vi "GLdrv_FILE_DRIVE.vi"(0 "Connection ID":T1, 11 "error in (no error)":errorcluster) -> (4 "Connection ID Out":T1, 6 "Drive out":string[](array[string]), 15 "error out":errorcluster)   [LabVIEW 2017, in "GL860_Driver.lvlib"]
doc: "認識されているデバイスを表示します\nMEM=内蔵メモリ\nSD=SDカード\n例) :FILE:DRIVE “MEM:HDD SD:HDD”"
uses:
  GL860_Driver.lvlib
  ConnectionID.ctl
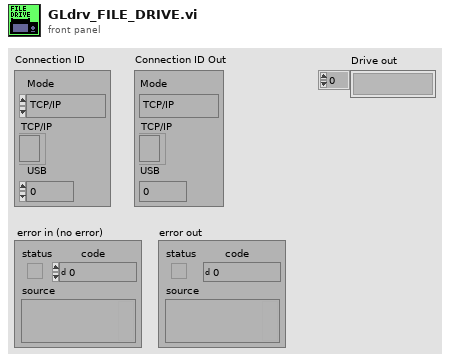
[diagram p1: front panel]
types:
  T1 = typedef "ConnectionID.ctl" = cluster{"Mode":enum16{"TCP/IP", "USB"}, "TCP/IP":refnum<k5>, "USB":i32}
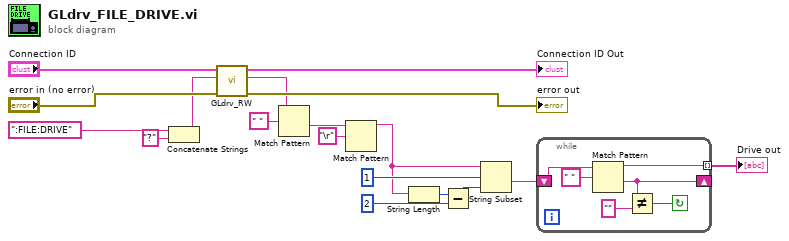
[diagram p0: block diagram]
diagram:
  n1 = Concatenate Strings(":FILE:DRIVE" ("Command"), "?" ("string")) -> (w9:string)
  n2 = call "GLdrv_RW.vi"("error in (no error)"="error in (no error)", "data in"=w9, "Connection ID"="Connection ID") -> ("error out"=→"error out":errorcluster, "data out"=w8:string, "Connection ID Out"=→"Connection ID Out":T1)  [unwired: 4 in, 2 out]
  n3 = Match Pattern(string=w8, regular expression=" " ("search string/char (-)")) -> (after substring=w11:string)  [unwired: 4 out]
  n4 = Match Pattern(string=w11, regular expression="\r") -> (before substring=w3:string)  [unwired: 4 out]
  n5 = String Length(string=w3) -> (length=w5:i32)
  n6 = Subtract(x=w5, y=2) -> (x-y=w6:i32)
  n7 = String Subset(string=w3, offset (0)=1, length (rest)=w6) -> (substring=w2:string)
  n8 = while {
    shift-right: [w22] -> _
    shift-left: w2 -> [w24]
    tunnel: [w23] -> w1 mode=indexing
    stop <- w19 continue-if-true
    n9 = Match Pattern(string=w24, regular expression=" ") -> (before substring=w23:string, after substring=w22:string)  [unwired: 3 out]
    n10 = Not Equal?(x=w22, y="") -> (x != y?=w19:bool)
  }
  "Drive out" <- w1
